vi "Read_all_waveforms.vi"(0 "tdms file in":refnum<k34>, 1 "error in":errorcluster, 3 "Channel names":string[](array[string]), 4 "Group name":string, 5 "Intensity_in":i32[][](array[numeric]), 6 "Peak_data_in":T2, 7 "In_cluster":cluster{"X_in":dbl[], "Y_in":dbl[]}) -> (12 "Peak_data_out":T2, 13 "Out_Cluster":T1, 14 "tdms file out":refnum<k34>, 15 "error out":errorcluster, 17 "Waveforms":waveform(dbl)[](array[waveform]), 18 "Spectrum":T3(array[cluster]), 19 "Intensity_out":i32[][](array[numeric]))   [LabVIEW 2019]
uses:
  SiPM_Tests_Global_Var.vi
  Agilent_lib/Agilent 2000 3000 X-Series.lvlib
  <vilib>/Analysis/NI_AALPro.lvlib
  <vilib>/gmath/NI_Gmath.lvlib
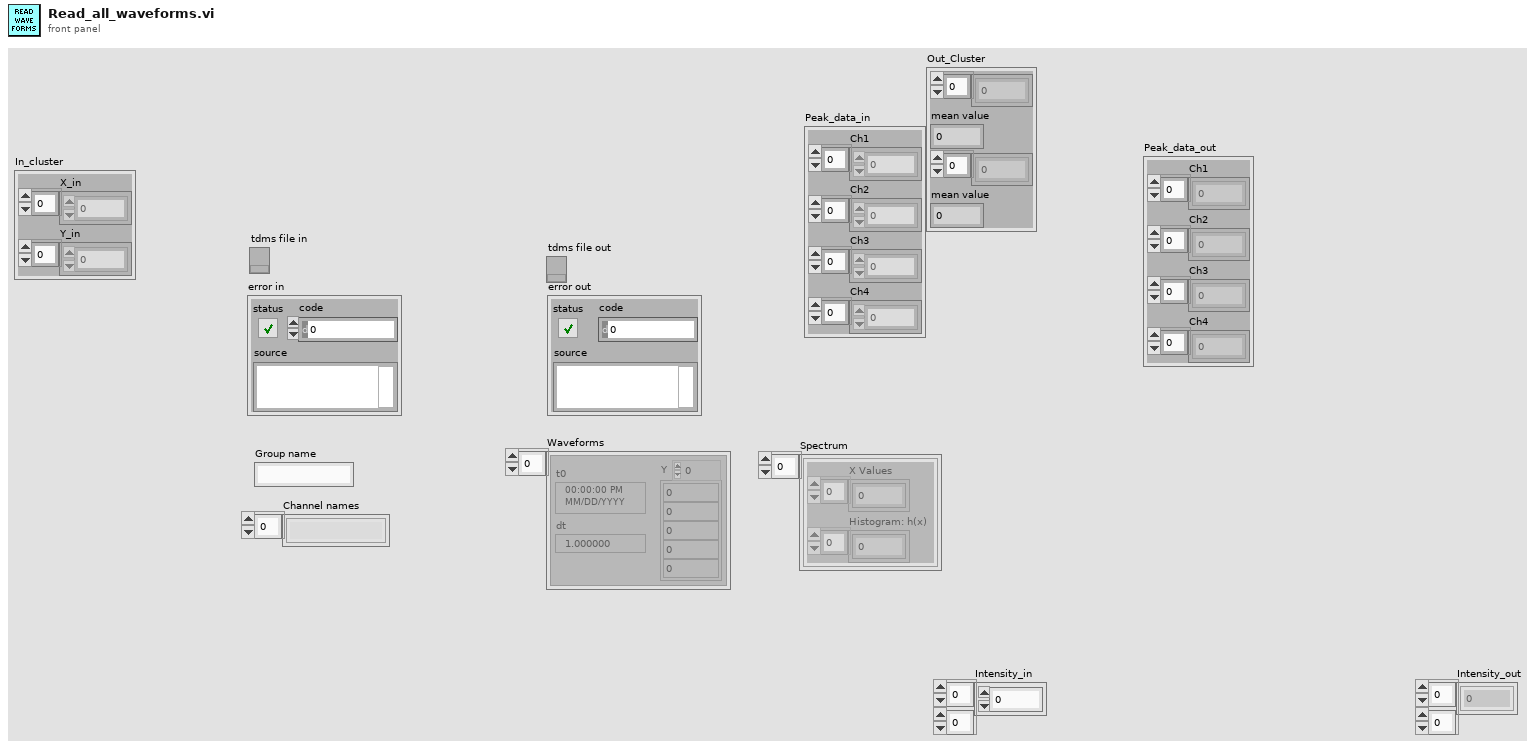
[diagram p1: front panel]
types:
  T1 = cluster{dbl[], "mean value":dbl, dbl[], "mean value":dbl}
  T2 = cluster{"Ch1":dbl[], "Ch2":dbl[], "Ch3":dbl[], "Ch4":dbl[]}
  T3 = cluster{"X Values":dbl[], "Histogram: h(x)":i32[]}[]
  T4 = cluster{"X Values":dbl[], "Histogram: h(x)":i32[]}
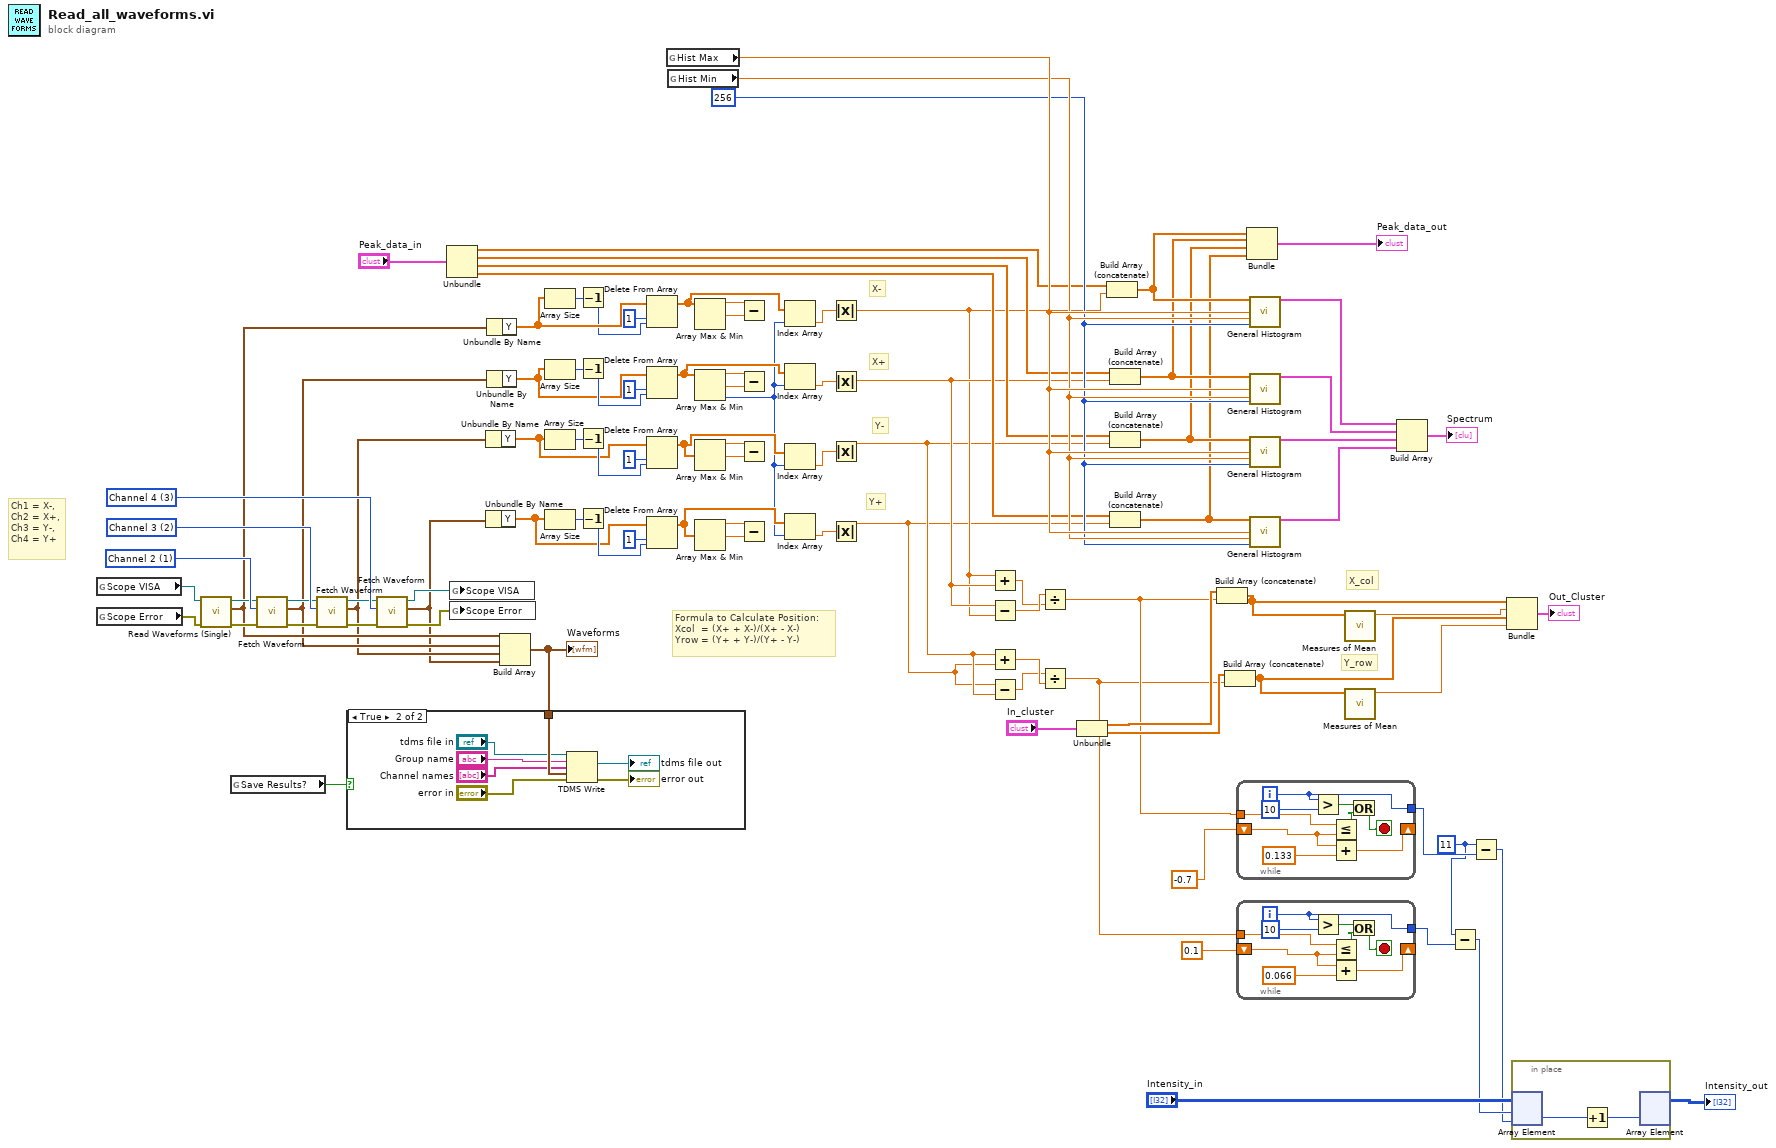
[diagram p0: block diagram]
diagram:
  w9 = 11 ("x")
  w52 = 256 ("# bins")
  w94 = 3 items=["Channel 1"=0, "Channel 2"=1, "Channel 3"=2, "Channel 4"=3, "Waveform Memory 1"=5, "Waveform Memory 2"=6, "Serial Bus 1"=7, "Serial Bus 2"=8, "Digital Bus Low"=9, "Digital Bus High "=10, "Digital Bus 1"=11, "Digital Bus 2"=12, "Function 1"=32, "Function 2"=33, "Function 3"=34, "Function 4"=35, "Math 1"=36, "Math 2"=37, "Math 3"=38, "Math 4"=39] ("Source Channel (0: Channel 1)")
  w96 = 2 items=["Channel 1"=0, "Channel 2"=1, "Channel 3"=2, "Channel 4"=3, "Waveform Memory 1"=5, "Waveform Memory 2"=6, "Serial Bus 1"=7, "Serial Bus 2"=8, "Digital Bus Low"=9, "Digital Bus High "=10, "Digital Bus 1"=11, "Digital Bus 2"=12, "Function 1"=32, "Function 2"=33, "Function 3"=34, "Function 4"=35, "Math 1"=36, "Math 2"=37, "Math 3"=38, "Math 4"=39] ("Source Channel (0: Channel 1)")
  w97 = 1 items=["Channel 1"=0, "Channel 2"=1, "Channel 3"=2, "Channel 4"=3, "Waveform Memory 1"=5, "Waveform Memory 2"=6, "Serial Bus 1"=7, "Serial Bus 2"=8, "Digital Bus Low"=9, "Digital Bus High "=10, "Digital Bus 1"=11, "Digital Bus 2"=12, "Function 1"=32, "Function 2"=33, "Function 3"=34, "Function 4"=35, "Math 1"=36, "Math 2"=37, "Math 3"=38, "Math 4"=39] ("Source Channel (0: Channel 1)")
  # "Y_row"
  # "X_col"
  # "Formula to Calculate Position:\nXcol  = (X+ + X-)/(X+ - X-)\nYrow = (Y+ + Y-)/(Y+ - Y-)"
  # "Y+"
  # "Y-"
  # "X+"
  # "X-"
  # "Ch1 = X-,\nCh2 = X+,\nCh3 = Y-,\nCh4 = Y+"
  n1 = global read "SiPM_Tests_Global_Var.vi" "Scope VISA"() -> (w86:refnum<visa-resource-name>)
  n2 = global read "SiPM_Tests_Global_Var.vi" "Scope Error"() -> (w87:errorcluster)
  n3 = call "Read Waveforms (Single).vi"("error in (no error)"=w87, "VISA resource name"=w86) -> ("error out"=w89:errorcluster, "Waveform Data"=w83:waveform(dbl), "VISA resource name out"=w88:refnum<visa-resource-name>)  [unwired: 7 in]
  n4 = global read "SiPM_Tests_Global_Var.vi" "Save Results?"() -> (w42:bool)
  n5 = call "Fetch Waveform.vi"("error in (no error)"=w89, "Source Channel (0: Channel 1)"=w97, "VISA resource name"=w88) -> ("error out"=w91:errorcluster, "Waveform Data"=w82:waveform(dbl), "VISA resource name out"=w90:refnum<visa-resource-name>)  [unwired: 2 in, 4 out]
  n6 = call "Fetch Waveform.vi"("error in (no error)"=w91, "Source Channel (0: Channel 1)"=w96, "VISA resource name"=w90) -> ("error out"=w93:errorcluster, "Waveform Data"=w81:waveform(dbl), "VISA resource name out"=w92:refnum<visa-resource-name>)  [unwired: 2 in, 4 out]
  n7 = call "Fetch Waveform.vi"("error in (no error)"=w93, "Source Channel (0: Channel 1)"=w94, "VISA resource name"=w92) -> ("error out"=w84:errorcluster, "Waveform Data"=w55:waveform(dbl), "VISA resource name out"=w85:refnum<visa-resource-name>)  [unwired: 2 in, 4 out]
  n8 = Unbundle("Peak_data_in") -> ("Ch1"=w49:dbl[], "Ch2"=w48:dbl[], "Ch3"=w47:dbl[], "Ch4"=w46:dbl[])
  n9 = global write "SiPM_Tests_Global_Var.vi" "Scope VISA"(w85) -> ()
  n10 = global write "SiPM_Tests_Global_Var.vi" "Scope Error"(w84) -> ()
  n11 = Unbundle By Name(w81) -> ("Y"=w44:dbl[])
  n12 = Unbundle By Name(w55) -> ("Y"=w43:dbl[])
  n13 = Unbundle By Name(w83) -> ("Y"=w75:dbl[])
  n14 = Unbundle By Name(w82) -> ("Y"=w67:dbl[])
  n15 = Build Array(w83, w82, w81, w55) -> (w95:waveform(dbl)[])
  "Waveforms" <- w95
  n16 = case shown="True" w42 {
    tunnel: w95 -> [_ w104]
    frame False {
    }
    frame True {
      n17 = TDMS Write(0:"tdms file in", 5:"Group name", 7:"Channel names", 9:w104, 11:"error in") -> (4:→"tdms file out":refnum<k34>, 15:→"error out":errorcluster)  [unwired: 1 in, 2 out]
    }
  }
  n18 = Array Size(array=w75) -> (size(s)=w74:i32)
  n19 = Array Size(array=w67) -> (size(s)=w71:i32)
  n20 = Array Size(array=w44) -> (size(s)=w63:i32)
  n21 = Array Size(array=w43) -> (size(s)=w58:i32)
  n22 = Decrement(x=w74) -> (x-1=w73:i32)
  n23 = Decrement(x=w71) -> (x-1=w72:i32)
  n24 = Decrement(x=w63) -> (x-1=w62:i32)
  n25 = Decrement(x=w58) -> (x-1=w59:i32)
  n26 = Delete From Array(array=w75, length=1, index=w73) -> (array with subset deleted=w21:dbl[])  [unwired: 1 out]
  n27 = Delete From Array(array=w67, length=1, index=w72) -> (array with subset deleted=w18:dbl[])  [unwired: 1 out]
  n28 = Delete From Array(array=w44, length=1, index=w62) -> (array with subset deleted=w16:dbl[])  [unwired: 1 out]
  n29 = Delete From Array(array=w43, length=1, index=w59) -> (array with subset deleted=w3:dbl[])  [unwired: 1 out]
  n30 = global read "SiPM_Tests_Global_Var.vi" "Hist Max"() -> (w54:dbl)
  n31 = global read "SiPM_Tests_Global_Var.vi" "Hist Min"() -> (w53:dbl)
  n32 = Array Max & Min(array=w21) -> (max value=w80:dbl, min value=w79:dbl)  [unwired: 2 out]
  n33 = Array Max & Min(array=w18) -> (max value=w68:dbl, min value=w69:dbl, min index (indices)=w2:i32)  [unwired: 1 out]
  n34 = Array Max & Min(array=w16) -> (max value=w66:dbl, min value=w65:dbl)  [unwired: 2 out]
  n35 = Array Max & Min(array=w3) -> (max value=w56:dbl, min value=w20:dbl)  [unwired: 2 out]
  n36 = Subtract(x=w80, y=w79) -> ()  [unwired: 1 out]
  n37 = Subtract(x=w68, y=w69) -> ()  [unwired: 1 out]
  n38 = Subtract(x=w66, y=w65) -> ()  [unwired: 1 out]
  n39 = Subtract(x=w56, y=w20) -> ()  [unwired: 1 out]
  n40 = Index Array(array=w21, index=w2) -> (element=w19:dbl)
  n41 = Index Array(array=w18, index=w2) -> (element=w1:dbl)
  n42 = Index Array(array=w16, index=w2) -> (element=w17:dbl)
  n43 = Index Array(array=w3, index=w2) -> (element=w4:dbl)
  n44 = Absolute Value(x=w19) -> (abs(x)=w40:dbl)
  n45 = Absolute Value(x=w1) -> (abs(x)=w41:dbl)
  n46 = Absolute Value(x=w17) -> (abs(x)=w39:dbl)
  n47 = Absolute Value(x=w4) -> (abs(x)=w38:dbl)
  n48 = Add(x=w40, y=w41) -> (x+y=w32:dbl)
  n49 = Subtract(x=w41, y=w40) -> (x-y=w33:dbl)
  n50 = Add(x=w39, y=w38) -> (x+y=w31:dbl)
  n51 = Subtract(x=w38, y=w39) -> (x-y=w30:dbl)
  n52 = Divide(x=w33, y=w32) -> (x/y=w6:dbl)
  n53 = Divide(x=w30, y=w31) -> (x/y=w5:dbl)
  n54 = Unbundle("In_cluster") -> ("X_in"=w23:dbl[], "Y_in"=w22:dbl[])
  n55 = Build Array (concatenate)(w49, w40) -> (w37:dbl[])
  n56 = Build Array (concatenate)(w48, w41) -> (w36:dbl[])
  n57 = Build Array (concatenate)(w47, w39) -> (w35:dbl[])
  n58 = Build Array (concatenate)(w46, w38) -> (w34:dbl[])
  n59 = Build Array (concatenate)(w23, w6) -> (w29:dbl[])
  n60 = Build Array (concatenate)(w22, w5) -> (w27:dbl[])
  n61 = while {
    tunnel: w6 -> [w113]
    shift-right: [w111] -> _
    shift-left: -0.7 ("y") -> [w112]
    tunnel: [w106] -> w11
    i -> [w106]
    stop <- w109 stop-if-true
    n62 = Greater?(x=w106, y=10) -> (0:w107:bool)
    n63 = Less Or Equal?(x=w113, y=w112) -> (x <= y?=w108:bool)
    n64 = Add(x=w112, y=0.133) -> (x+y=w111:dbl)
    n65 = Or(x=w107, y=w108) -> (x .or. y?=w109:bool)
  }
  n66 = while {
    tunnel: w5 -> [w122]
    shift-right: [w120] -> _
    shift-left: 0.1 ("y") -> [w121]
    tunnel: [w115] -> w10
    i -> [w115]
    stop <- w118 stop-if-true
    n67 = Greater?(x=w115, y=10) -> (0:w116:bool)
    n68 = Less Or Equal?(x=w122, y=w121) -> (x <= y?=w117:bool)
    n69 = Add(x=w121, y=0.066) -> (x+y=w120:dbl)
    n70 = Or(x=w116, y=w117) -> (x .or. y?=w118:bool)
  }
  n71 = Bundle(w37, w36, w35, w34) -> (→"Peak_data_out":cluster{dbl[], dbl[], dbl[], dbl[]})  [unwired: 1 in]
  n72 = call <vilib>:"General Histogram.vi"("X"=w37, "max"=w54, "min"=w53, "# bins"=w52) -> ("Histogram Graph"=w78:T4)  [unwired: 7 in, 4 out]
  n73 = call <vilib>:"General Histogram.vi"("X"=w36, "max"=w54, "min"=w53, "# bins"=w52) -> ("Histogram Graph"=w61:T4)  [unwired: 7 in, 4 out]
  n74 = call <vilib>:"General Histogram.vi"("X"=w35, "max"=w54, "min"=w53, "# bins"=w52) -> ("Histogram Graph"=w60:T4)  [unwired: 7 in, 4 out]
  n75 = call <vilib>:"General Histogram.vi"("X"=w34, "max"=w54, "min"=w53, "# bins"=w52) -> ("Histogram Graph"=w51:T4)  [unwired: 7 in, 4 out]
  n76 = call <vilib>:"Measures of Mean.vi"("x array"=w29) -> ("mean value"=w28:dbl)  [unwired: 9 in, 1 out]
  n77 = call <vilib>:"Measures of Mean.vi"("x array"=w27) -> ("mean value"=w26:dbl)  [unwired: 9 in, 1 out]
  n78 = Build Array(w78, w61, w60, w51) -> (→"Spectrum":T3)
  n79 = Subtract(x=w9, y=w10) -> (x-y=w8:i32)
  n80 = Subtract(x=w9, y=w11) -> (x-y=w7:i32)
  n81 = Bundle(w29, "mean value"=w28, w27, "mean value"=w26) -> (→"Out_Cluster":T1)  [unwired: 1 in]
  n82 = in-place {
    n83 = in-place-array #1("Intensity_in", w8, w7) -> (w124:i32)
    n84 = Increment(x=w124) -> (x+1=w123:i32)
    n85 = in-place-array #1(w123) -> (→"Intensity_out":i32[][])  [unwired: 2 out]
  }
